vi "XNET TCP Socket Open.vi"(4 "local interface":string, 6 "local port":u16, 7 "stack":refnum<k21>, 8 "error in":errorcluster, 9 "timeout ms (60000)":i32=60000, 10 "remote port":u16, 11 "remote address":string) -> (0 "error out":errorcluster, 3 "socket":refnum<k20>)   [LabVIEW 2018]
doc: "Opens a TCP network connection using a specified address and port."
uses:
  nixlvapi.dll
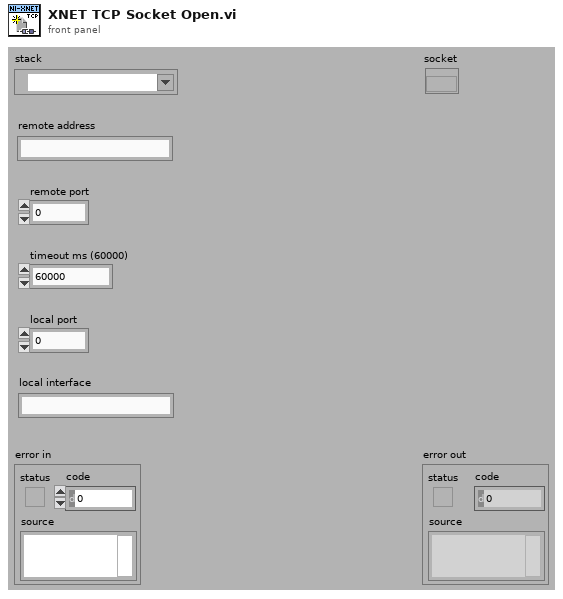
[diagram p1: front panel]
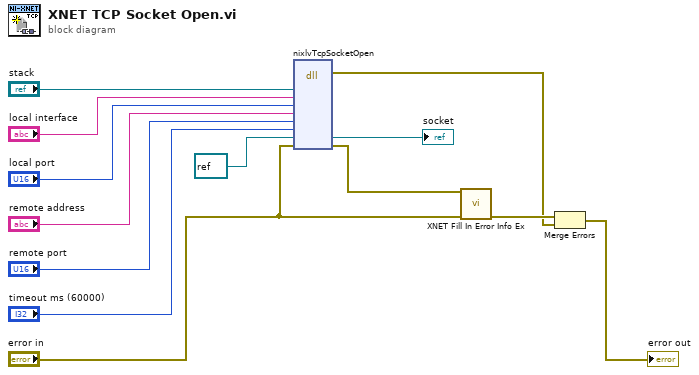
[diagram p0: block diagram]
diagram:
  n1 = dll-call lib="nixlvapi.*" fn="nixlvTcpSocketOpen" label="Call Library"("stackRef"="stack", "localInterface"="local interface", "localPort"="local port", "remoteAddress"="remote address", "remotePort"="remote port", "timeoutMs"="timeout ms (60000)", "socketRefObjPtr"=refnum<k20> refnum ("socket"), "errorInOut"="error in") -> (error out=w11:errorcluster, "socketRefObjPtr"=→"socket":refnum<k20>, "errorInOut"=w13:errorcluster)  [unwired: 3 in, 8 out]
  n2 = call "XNET Fill In Error Info Ex.vi"("error xnet"=w13, "error in"="error in") -> ("error out"=w12:errorcluster)  [unwired: 13 in]
  n3 = Merge Errors(w12, w11) -> (→"error out":errorcluster)
